vi "Init Log.vi"(8 "error in (no error)":errorcluster, 11 "S4GUI in":refnum<class "S4GUI.lvclass">) -> (0 "error out":errorcluster, 3 "S4GUI out":refnum<class "S4GUI.lvclass">)   [LabVIEW 2018, in "S4GUI.lvclass"]
uses:
  S4GUI.lvclass
  S4GUI.lvclass/S4GUI.ctl
  Log/Log.lvclass
  Acquisition/Acquisition.lvclass
  Instrument/Instrument.lvclass
  TCS/TCS.lvclass
  SyncBox/Sync Box.lvclass
  TelFocus/TelFocus.lvclass
  WeatherStation/WeatherStation.lvclass
  Comm/Stream/Stream.lvclass
panel:
  out "concatenated string":string
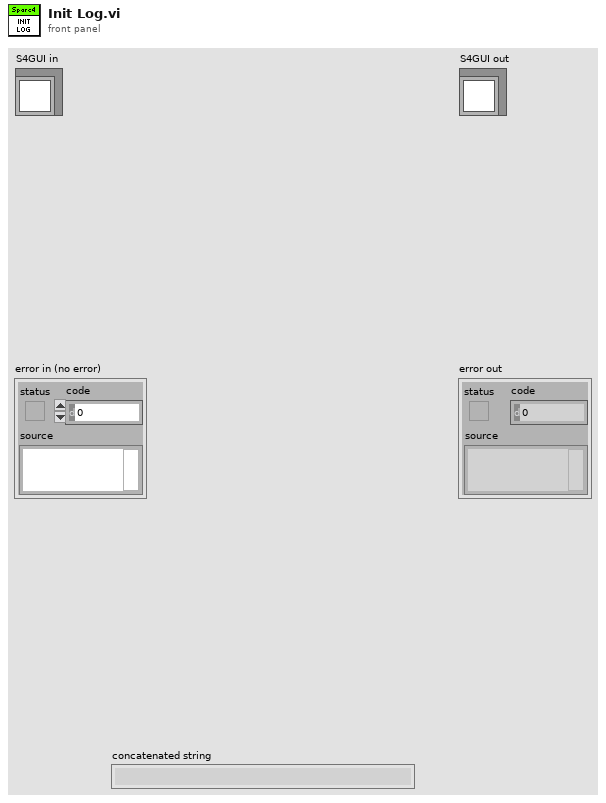
[diagram p1: front panel]
types:
  T1 = enum16{"open", "replace", "create", "open or create", "replace or create", "replace or create with confirmation"}
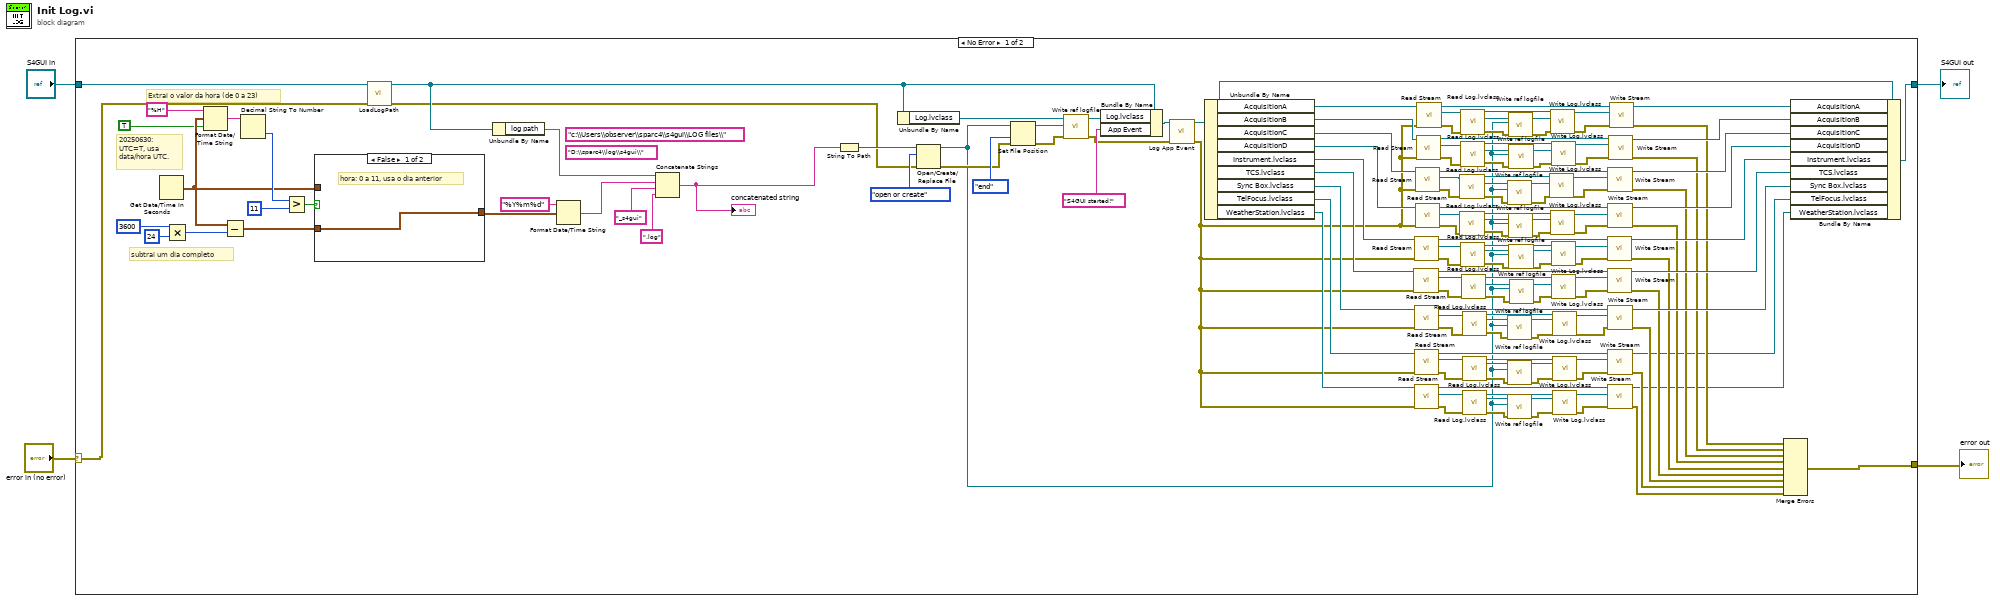
[diagram p0: block diagram]
diagram:
  n1 = case shown="No Error" "error in (no error)" {
    selector: "error in (no error)" -> [w7 w163]
    tunnel: [w134 w163] -> w3
    tunnel: [w156 w162] -> w1
    tunnel: "S4GUI in" -> [w9 w162]
    frame No Error {
      (unwired) "D:\\sparc4\\log\\s4gui\\" ("string")
      (unwired) "c:\\Users\\observer\\sparc4\\s4gui\\LOG files\\" ("string")
      # "20250630:\nUTC=T, usa\ndata/hora UTC."
      # "Extrai o valor da hora (de 0 a 23)"
      # "subtrai um dia completo"
      n2 = Get Date/Time In Seconds() -> (seconds since 1Jan1904=w37:timestamp)
      n3 = Multiply(x=3600, y=24) -> (x*y=w35:i32)
      n4 = Format Date/Time String(time format string (%c)="%H", seconds (now)=w37, UTC format=TRUE) -> (date/time string=w39:string)
      n5 = Subtract(x=w37, y=w35) -> (x-y=w34:timestamp)
      n6 = Decimal String To Number(string=w39) -> (number=w41:i32)  [unwired: 2 in, 1 out]
      n7 = Greater?(x=w41, y=11) -> (0:w40:bool)
      n8 = case shown="False" w40 {
        tunnel: w34 -> [w160 _]
        tunnel: w37 -> [_ w161]
        tunnel: [w160 w161] -> w38
        frame False {
          # "hora: 0 a 11, usa o dia anterior"
        }
        frame True {
          # "hora: 12 a 23, usa o dia atual."
        }
      }
      n9 = call-dynamic "LoadLogPath.vi"("error in (no error)"=w7, "S4GUI in"=w9) -> ("error out"=w6:errorcluster, "S4GUI out"=w8:refnum<class "S4GUI.lvclass">)  [unwired: 8 in]
      n10 = Unbundle By Name(w8) -> ("log path"=w10:string)
      n11 = Format Date/Time String(time format string (%c)="%Y%m%d", seconds (now)=w38) -> (date/time string=w36:string)  [unwired: 1 in]
      n12 = Concatenate Strings(w10, w36, "_s4gui" ("string"), ".log" ("string")) -> (w26:string)
      "concatenated string" <- w26
      n13 = String To Path(string=w26) -> (path=w158:path)
      n14 = Unbundle By Name(w8) -> ("Log.lvclass"=w64:refnum<class "Log.lvclass">)
      n15 = Open/Create/Replace File(file path (use dialog)=w158, error in=w6, operation (0:open)=T1."open or create") -> (refnum out=w12:refnum<file>, error out=w47:errorcluster)  [unwired: 3 in, 1 out]
      n16 = Set File Position(refnum=w12, from (0:start)=enum16{"start", "end", "current"}."end", error in=w47) -> (refnum out=w48:refnum<file>, error out=w46:errorcluster)  [unwired: 1 in]
      n17 = call-dynamic "Write ref logfile.vi"("error in (no error)"=w46, "ref logfile"=w48, "Log in"=w64) -> ("error out"=w43:errorcluster, "Log out"=w63:refnum<class "Log.lvclass">)  [unwired: 7 in]
      n18 = Bundle By Name(cluster=w8, "Log.lvclass"=w63, "App Event"="S4GUI started!") -> (w44:refnum<class "S4GUI.lvclass">)
      n19 = call-dynamic "Log App Event.vi"("error in (no error)"=w43, "S4GUI in"=w44) -> ("error out"=w11:errorcluster, "S4GUI out"=w42:refnum<class "S4GUI.lvclass">)  [unwired: 8 in]
      n20 = Unbundle By Name(w42) -> ("AcquisitionA"=w155:refnum<class "Acquisition.lvclass">, "AcquisitionB"=w154:refnum<class "Acquisition.lvclass">, "AcquisitionC"=w153:refnum<class "Acquisition.lvclass">, "AcquisitionD"=w152:refnum<class "Acquisition.lvclass">, "Instrument.lvclass"=w151:refnum<class "Instrument.lvclass">, "TCS.lvclass"=w150:refnum<class "TCS.lvclass">, "Sync Box.lvclass"=w149:refnum<class "Sync Box.lvclass">, "TelFocus.lvclass"=w55:refnum<class "TelFocus.lvclass">, "WeatherStation.lvclass"=w19:refnum<class "WeatherStation.lvclass">)
      n21 = call-dynamic "Read Stream.vi"("error in (no error)"=w11, "Server in"=w150) -> ("error out"=w70:errorcluster, "Stream.lvclass"=w71:refnum<class "Stream.lvclass">, "Server out"=w74:refnum<class "TCS.lvclass">)  [unwired: 7 in]
      n22 = call-dynamic "Read Stream.vi"("error in (no error)"=w11, "Server in"=w151) -> ("error out"=w86:errorcluster, "Stream.lvclass"=w88:refnum<class "Stream.lvclass">, "Server out"=w89:refnum<class "Instrument.lvclass">)  [unwired: 7 in]
      n23 = call-dynamic "Read Stream.vi"("error in (no error)"=w11, "Server in"=w149) -> ("error out"=w67:errorcluster, "Stream.lvclass"=w68:refnum<class "Stream.lvclass">, "Server out"=w69:refnum<class "Sync Box.lvclass">)  [unwired: 7 in]
      n24 = call-dynamic "Read Stream.vi"("error in (no error)"=w11, "Server in"=w55) -> ("error out"=w57:errorcluster, "Stream.lvclass"=w58:refnum<class "Stream.lvclass">, "Server out"=w54:refnum<class "TelFocus.lvclass">)  [unwired: 7 in]
      n25 = call-dynamic "Read Stream.vi"("error in (no error)"=w11, "Server in"=w19) -> ("error out"=w21:errorcluster, "Stream.lvclass"=w15:refnum<class "Stream.lvclass">, "Server out"=w16:refnum<class "WeatherStation.lvclass">)  [unwired: 7 in]
      n26 = call-dynamic "Read Stream.vi"("error in (no error)"=w11, "Server in"=w153) -> ("error out"=w101:errorcluster, "Stream.lvclass"=w103:refnum<class "Stream.lvclass">, "Server out"=w104:refnum<class "Acquisition.lvclass">)  [unwired: 7 in]
      n27 = call-dynamic "Read Stream.vi"("error in (no error)"=w11, "Server in"=w152) -> ("error out"=w96:errorcluster, "Stream.lvclass"=w95:refnum<class "Stream.lvclass">, "Server out"=w99:refnum<class "Acquisition.lvclass">)  [unwired: 7 in]
      n28 = call-dynamic "Read Stream.vi"("error in (no error)"=w11, "Server in"=w154) -> ("error out"=w119:errorcluster, "Stream.lvclass"=w118:refnum<class "Stream.lvclass">, "Server out"=w116:refnum<class "Acquisition.lvclass">)  [unwired: 7 in]
      n29 = call-dynamic "Read Stream.vi"("error in (no error)"=w11, "Server in"=w155) -> ("error out"=w129:errorcluster, "Stream.lvclass"=w133:refnum<class "Stream.lvclass">, "Server out"=w157:refnum<class "Acquisition.lvclass">)  [unwired: 7 in]
      n30 = call-dynamic "Read Log.lvclass.vi"("error in (no error)"=w101, "Comm in"=w103) -> ("error out"=w111:errorcluster, "Log.lvclass"=w114:refnum<class "Log.lvclass">, "Comm out"=w113:refnum<class "Stream.lvclass">)  [unwired: 7 in]
      n31 = call-dynamic "Read Log.lvclass.vi"("error in (no error)"=w96, "Comm in"=w95) -> ("error out"=w106:errorcluster, "Log.lvclass"=w109:refnum<class "Log.lvclass">, "Comm out"=w108:refnum<class "Stream.lvclass">)  [unwired: 7 in]
      n32 = call-dynamic "Read Log.lvclass.vi"("error in (no error)"=w129, "Comm in"=w133) -> ("error out"=w128:errorcluster, "Log.lvclass"=w132:refnum<class "Log.lvclass">, "Comm out"=w131:refnum<class "Stream.lvclass">)  [unwired: 7 in]
      n33 = call-dynamic "Read Log.lvclass.vi"("error in (no error)"=w119, "Comm in"=w118) -> ("error out"=w121:errorcluster, "Log.lvclass"=w124:refnum<class "Log.lvclass">, "Comm out"=w123:refnum<class "Stream.lvclass">)  [unwired: 7 in]
      n34 = call-dynamic "Read Log.lvclass.vi"("error in (no error)"=w86, "Comm in"=w88) -> ("error out"=w91:errorcluster, "Log.lvclass"=w94:refnum<class "Log.lvclass">, "Comm out"=w93:refnum<class "Stream.lvclass">)  [unwired: 7 in]
      n35 = call-dynamic "Read Log.lvclass.vi"("error in (no error)"=w70, "Comm in"=w71) -> ("error out"=w81:errorcluster, "Log.lvclass"=w84:refnum<class "Log.lvclass">, "Comm out"=w83:refnum<class "Stream.lvclass">)  [unwired: 7 in]
      n36 = call-dynamic "Read Log.lvclass.vi"("error in (no error)"=w67, "Comm in"=w68) -> ("error out"=w76:errorcluster, "Log.lvclass"=w79:refnum<class "Log.lvclass">, "Comm out"=w78:refnum<class "Stream.lvclass">)  [unwired: 7 in]
      n37 = call-dynamic "Read Log.lvclass.vi"("error in (no error)"=w57, "Comm in"=w58) -> ("error out"=w60:errorcluster, "Log.lvclass"=w62:refnum<class "Log.lvclass">, "Comm out"=w52:refnum<class "Stream.lvclass">)  [unwired: 7 in]
      n38 = call-dynamic "Read Log.lvclass.vi"("error in (no error)"=w21, "Comm in"=w15) -> ("error out"=w23:errorcluster, "Log.lvclass"=w25:refnum<class "Log.lvclass">, "Comm out"=w14:refnum<class "Stream.lvclass">)  [unwired: 7 in]
      n39 = call-dynamic "Write ref logfile.vi"("error in (no error)"=w111, "ref logfile"=w12, "Log in"=w114) -> ("error out"=w110:errorcluster, "Log out"=w112:refnum<class "Log.lvclass">)  [unwired: 7 in]
      n40 = call-dynamic "Write ref logfile.vi"("error in (no error)"=w76, "ref logfile"=w12, "Log in"=w79) -> ("error out"=w75:errorcluster, "Log out"=w77:refnum<class "Log.lvclass">)  [unwired: 7 in]
      n41 = call-dynamic "Write ref logfile.vi"("error in (no error)"=w60, "ref logfile"=w12, "Log in"=w62) -> ("error out"=w59:errorcluster, "Log out"=w61:refnum<class "Log.lvclass">)  [unwired: 7 in]
      n42 = call-dynamic "Write ref logfile.vi"("error in (no error)"=w23, "ref logfile"=w12, "Log in"=w25) -> ("error out"=w22:errorcluster, "Log out"=w24:refnum<class "Log.lvclass">)  [unwired: 7 in]
      n43 = call-dynamic "Write ref logfile.vi"("error in (no error)"=w128, "ref logfile"=w12, "Log in"=w132) -> ("error out"=w127:errorcluster, "Log out"=w130:refnum<class "Log.lvclass">)  [unwired: 7 in]
      n44 = call-dynamic "Write ref logfile.vi"("error in (no error)"=w106, "ref logfile"=w12, "Log in"=w109) -> ("error out"=w105:errorcluster, "Log out"=w107:refnum<class "Log.lvclass">)  [unwired: 7 in]
      n45 = call-dynamic "Write ref logfile.vi"("error in (no error)"=w121, "ref logfile"=w12, "Log in"=w124) -> ("error out"=w120:errorcluster, "Log out"=w122:refnum<class "Log.lvclass">)  [unwired: 7 in]
      n46 = call-dynamic "Write ref logfile.vi"("error in (no error)"=w91, "ref logfile"=w12, "Log in"=w94) -> ("error out"=w90:errorcluster, "Log out"=w92:refnum<class "Log.lvclass">)  [unwired: 7 in]
      n47 = call-dynamic "Write ref logfile.vi"("error in (no error)"=w81, "ref logfile"=w12, "Log in"=w84) -> ("error out"=w80:errorcluster, "Log out"=w82:refnum<class "Log.lvclass">)  [unwired: 7 in]
      n48 = call-dynamic "Write Log.lvclass.vi"("error in (no error)"=w110, "Log.lvclass"=w112, "Comm in"=w113) -> ("error out"=w100:errorcluster, "Comm out"=w102:refnum<class "Stream.lvclass">)  [unwired: 7 in]
      n49 = call-dynamic "Write Log.lvclass.vi"("error in (no error)"=w127, "Log.lvclass"=w130, "Comm in"=w131) -> ("error out"=w126:errorcluster, "Comm out"=w125:refnum<class "Stream.lvclass">)  [unwired: 7 in]
      n50 = call-dynamic "Write Log.lvclass.vi"("error in (no error)"=w105, "Log.lvclass"=w107, "Comm in"=w108) -> ("error out"=w97:errorcluster, "Comm out"=w98:refnum<class "Stream.lvclass">)  [unwired: 7 in]
      n51 = call-dynamic "Write Log.lvclass.vi"("error in (no error)"=w120, "Log.lvclass"=w122, "Comm in"=w123) -> ("error out"=w115:errorcluster, "Comm out"=w117:refnum<class "Stream.lvclass">)  [unwired: 7 in]
      n52 = call-dynamic "Write Log.lvclass.vi"("error in (no error)"=w90, "Log.lvclass"=w92, "Comm in"=w93) -> ("error out"=w85:errorcluster, "Comm out"=w87:refnum<class "Stream.lvclass">)  [unwired: 7 in]
      n53 = call-dynamic "Write Log.lvclass.vi"("error in (no error)"=w80, "Log.lvclass"=w82, "Comm in"=w83) -> ("error out"=w72:errorcluster, "Comm out"=w73:refnum<class "Stream.lvclass">)  [unwired: 7 in]
      n54 = call-dynamic "Write Log.lvclass.vi"("error in (no error)"=w75, "Log.lvclass"=w77, "Comm in"=w78) -> ("error out"=w66:errorcluster, "Comm out"=w65:refnum<class "Stream.lvclass">)  [unwired: 7 in]
      n55 = call-dynamic "Write Log.lvclass.vi"("error in (no error)"=w59, "Log.lvclass"=w61, "Comm in"=w52) -> ("error out"=w56:errorcluster, "Comm out"=w51:refnum<class "Stream.lvclass">)  [unwired: 7 in]
      n56 = call-dynamic "Write Log.lvclass.vi"("error in (no error)"=w22, "Log.lvclass"=w24, "Comm in"=w14) -> ("error out"=w20:errorcluster, "Comm out"=w13:refnum<class "Stream.lvclass">)  [unwired: 7 in]
      n57 = call-dynamic "Write Stream.vi"("error in (no error)"=w85, "Stream.lvclass"=w87, "Server in"=w89) -> ("error out"=w137:errorcluster, "Server out"=w144:refnum<class "Instrument.lvclass">)  [unwired: 7 in]
      n58 = call-dynamic "Write Stream.vi"("error in (no error)"=w72, "Stream.lvclass"=w73, "Server in"=w74) -> ("error out"=w136:errorcluster, "Server out"=w143:refnum<class "TCS.lvclass">)  [unwired: 7 in]
      n59 = call-dynamic "Write Stream.vi"("error in (no error)"=w100, "Stream.lvclass"=w102, "Server in"=w104) -> ("error out"=w139:errorcluster, "Server out"=w146:refnum<class "Acquisition.lvclass">)  [unwired: 7 in]
      n60 = call-dynamic "Write Stream.vi"("error in (no error)"=w97, "Stream.lvclass"=w98, "Server in"=w99) -> ("error out"=w138:errorcluster, "Server out"=w145:refnum<class "Acquisition.lvclass">)  [unwired: 7 in]
      n61 = call-dynamic "Write Stream.vi"("error in (no error)"=w66, "Stream.lvclass"=w65, "Server in"=w69) -> ("error out"=w135:errorcluster, "Server out"=w142:refnum<class "Sync Box.lvclass">)  [unwired: 7 in]
      n62 = call-dynamic "Write Stream.vi"("error in (no error)"=w56, "Stream.lvclass"=w51, "Server in"=w54) -> ("error out"=w50:errorcluster, "Server out"=w53:refnum<class "TelFocus.lvclass">)  [unwired: 7 in]
      n63 = call-dynamic "Write Stream.vi"("error in (no error)"=w20, "Stream.lvclass"=w13, "Server in"=w16) -> ("error out"=w18:errorcluster, "Server out"=w17:refnum<class "WeatherStation.lvclass">)  [unwired: 7 in]
      n64 = call-dynamic "Write Stream.vi"("error in (no error)"=w115, "Stream.lvclass"=w117, "Server in"=w116) -> ("error out"=w140:errorcluster, "Server out"=w147:refnum<class "Acquisition.lvclass">)  [unwired: 7 in]
      n65 = call-dynamic "Write Stream.vi"("error in (no error)"=w126, "Stream.lvclass"=w125, "Server in"=w157) -> ("error out"=w141:errorcluster, "Server out"=w148:refnum<class "Acquisition.lvclass">)  [unwired: 7 in]
      n66 = Merge Errors(w141, w140, w139, w138, w137, w136, w135, w50, w18) -> (w134:errorcluster)
      n67 = Bundle By Name(cluster=w42, "AcquisitionA"=w148, "AcquisitionB"=w147, "AcquisitionC"=w146, "AcquisitionD"=w145, "Instrument.lvclass"=w144, "TCS.lvclass"=w143, "Sync Box.lvclass"=w142, "TelFocus.lvclass"=w53, "WeatherStation.lvclass"=w17) -> (w156:refnum<class "S4GUI.lvclass">)
    }
    frame Error {
    }
  }
  "error out" <- w3
  "S4GUI out" <- w1
